vi "Cal.vi"(8 "error in (no error)":errorcluster, 9 "b":dbl, 10 "a":dbl, 11 "Subtract in":refnum<class "Subtract.lvclass">) -> (0 "error out":errorcluster, 2 "Result":dbl, 3 "Subtract out":refnum<class "Subtract.lvclass">)   [LabVIEW 2014, in "Caculator.lvlib" / "Subtract.lvclass"]
uses:
  Subtract.lvclass
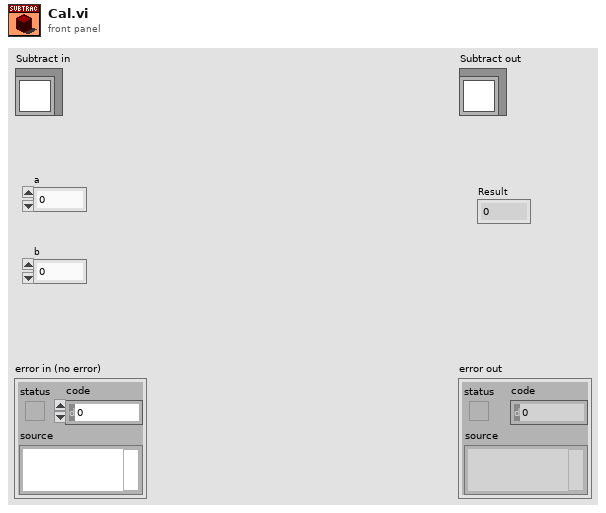
[diagram p1: front panel]
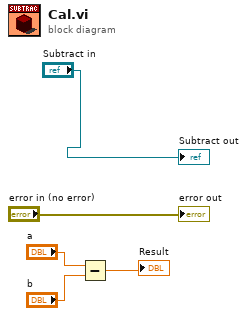
[diagram p0: block diagram]
diagram:
  n1 = Subtract(x="a", y="b") -> (x-y=→"Result":dbl)
  "error out" <- "error in (no error)"
  "Subtract out" <- "Subtract in"
